vi "Configure System (Date).vi"(8 "error in (no error)":errorcluster, 10 "Time Stamp":timestamp=timestamp(3250429200 s since 1904-01-01), 11 "VISA resource name":refnum<visa-resource-name>) -> (0 "error out":errorcluster, 3 "VISA resource name out":refnum<visa-resource-name>)   [LabVIEW 2016, in "Agilent E4980.lvlib"]
doc: "Sets the system date and time of the instrument."
uses:
  <instrlib>/Agilent E4980/Agilent E4980.lvlib
  <vilib>/regexp/Match Regular Expression.xnode
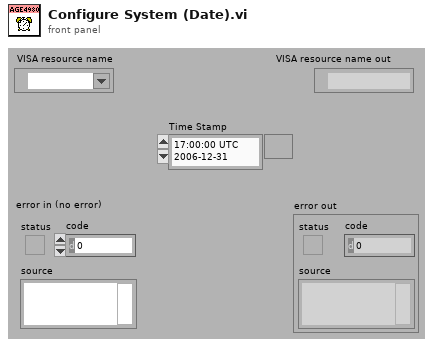
[diagram p1: front panel]
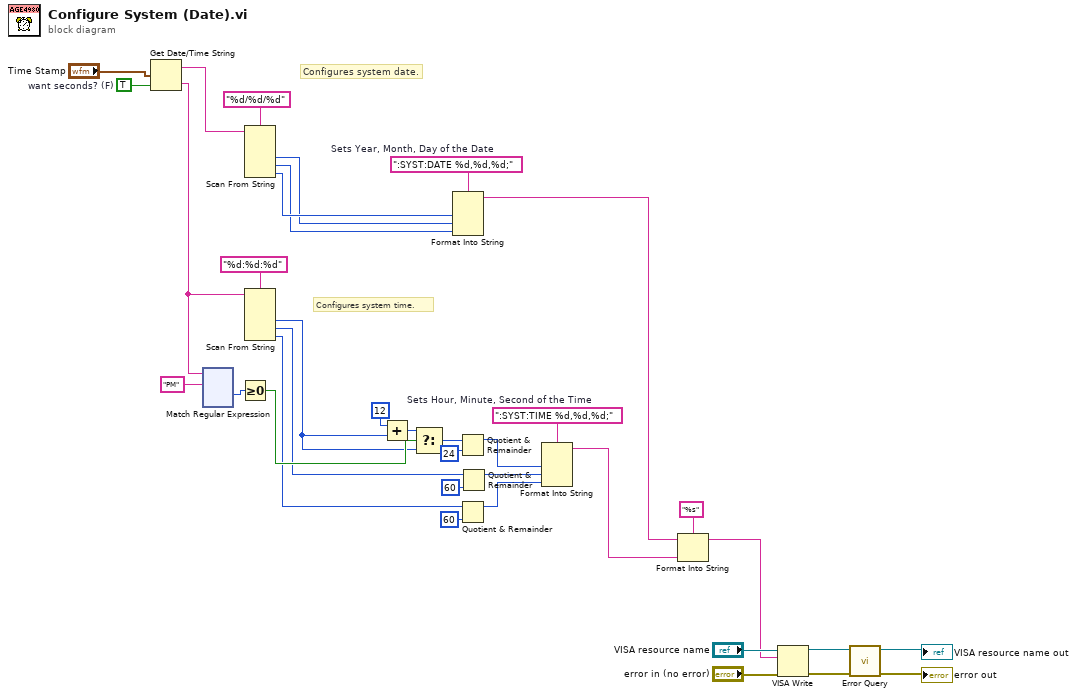
[diagram p0: block diagram]
diagram:
  w18 = ":SYST:TIME %d,%d,%d;"  # Sets Hour, Minute, Second of the Time
  w28 = TRUE  # want seconds? (F)
  w36 = ":SYST:DATE %d,%d,%d;"  # Sets Year, Month, Day of the Date
  # "Configures system time."
  # "Configures system date."
  n1 = Get Date/Time String(seconds (now)="Time Stamp", want seconds? (F)=w28) -> (date string=w26:string, time string=w6:string)  [unwired: 1 in]
  n2 = xnode "Match Regular Expression"("input string"=w6, "regular expression"="PM" ("format string")) -> ("offset past match"=w4:i32)  [unwired: 4 in, 4 out]
  n3 = Greater Or Equal To 0?(x=w4) -> (x >= 0?=w24:bool)
  n4 = Scan From String(format string="%d/%d/%d", input string=w26) -> (output 1=w2:i32, output 2=w1:i32, output 3=w3:i32)  [unwired: 5 in, 3 out]
  n5 = Scan From String(format string="%d:%d:%d", input string=w6) -> (output 1=w23:i32, output 2=w16:i32, output 3=w12:i32)  [unwired: 5 in, 3 out]
  n6 = Add(x=12, y=w23) -> (x+y=w21:i32)
  n7 = Select(t=w21, s=w24, f=w23) -> (s? t:f=w20:i32)
  n8 = Format Into String(format string=w36, w3, w2, w1) -> (resulting string=w9:string)  [unwired: 2 in, 1 out]
  n9 = Quotient & Remainder(x=w20, y=24) -> (x-y*floor(x/y)=w17:i32)  [unwired: 1 out]
  n10 = Quotient & Remainder(x=w12, y=60) -> (x-y*floor(x/y)=w11:i32)  [unwired: 1 out]
  n11 = Quotient & Remainder(x=w16, y=60) -> (x-y*floor(x/y)=w14:i32)  [unwired: 1 out]
  n12 = Format Into String(format string=w18, w17, w14, w11) -> (resulting string=w8:string)  [unwired: 2 in, 1 out]
  n13 = Format Into String(format string="%s", initial string=w9, w8) -> (resulting string=w7:string)  [unwired: 1 in, 1 out]
  n14 = VISA Write(VISA resource name="VISA resource name", write buffer=w7, error in (no error)="error in (no error)") -> (VISA resource name out=w33:refnum<visa-resource-name>, error out=w32:errorcluster)  [unwired: 1 out]
  n15 = call <instrlib>:"Error Query.vi"("error in (no error)"=w32, "VISA resource name"=w33) -> ("error out"=→"error out":errorcluster, "VISA resource name out"=→"VISA resource name out":refnum<visa-resource-name>)  [unwired: 6 in, 2 out]
